vi "ExtendedKalmanFilter_SetXHat.vi"(10 "xHat":T1, 11 "in ExtendedKalmanFiilter":T2) -> (0 "Size Coerced":bool, 3 "out ExtendedKalmanFiilter":T2)   [LabVIEW 2019, in "Trajectory_Library.lvlib"]
doc: "Set initial state estimate x-hat.\n \nInputs:\n - inExtendedKalmanFIlter -- filter data cluster\n - xHat The state estimate x-hat.\n\nReturns:\n - outExtendedKalmanFIlter -- updated filter data cluster\n - sizeCoerced -- If TRUE, an unexpected error occured."
uses:
  Trajectory_Library.lvlib
  TypeDef/EXTENDED_KALMAN_FILTER.ctl
  <vilib>/Analysis/Matrix/Datatypes/RealMatrix.ctl
  MatBuilder_Create.vi
  <vilib>/Analysis/Matrix/NI_Matrix.lvlib
panel:
  # "State Estimate <Statess,1>"
  # "<States, States>"
  # "<States, States>"
  # "<Statess,  States>"
  # "<Outputs, Outputs>"
  # "State Estimate <Statess,1>"
  # "<States, States>"
  # "<States, States>"
  # "<Statess,  States>"
  # "<Outputs, Outputs>"
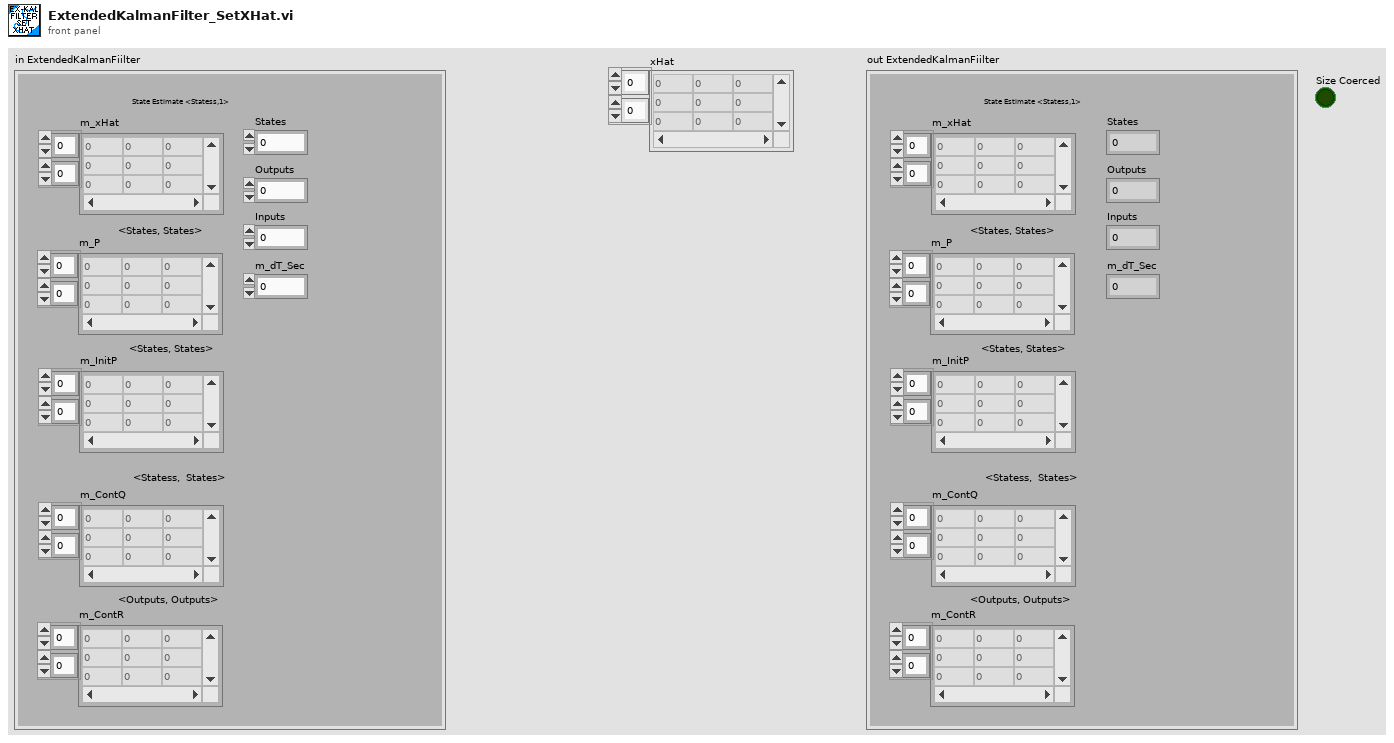
[diagram p1: front panel]
types:
  T1 = typedef "NI_Matrix.lvlib/RealMatrix.ctl" = dbl[][]
  T2 = typedef "Trajectory_Library.lvlib/EXTENDED_KALMAN_FILTER.ctl" = cluster{"m_P":T1, "m_xHat":T1, "States":i32, "Outputs":i32, "m_ContR":T1, "m_ContQ":T1, "m_dT_Sec":dbl, "Inputs":i32, "m_InitP":T1}
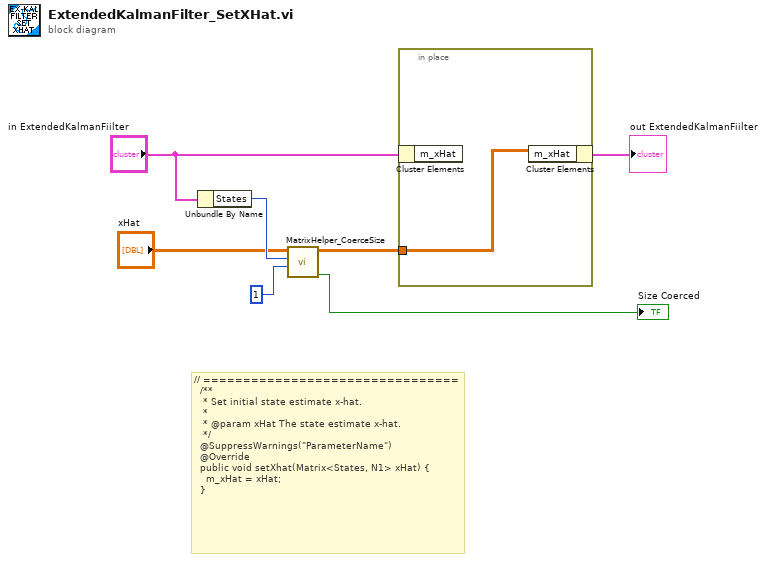
[diagram p0: block diagram]
diagram:
  # "// ================================\n  /**\n   * Set initial state estimate x-hat.\n   *\n   * @param xHat The state estimate x-hat.\n   */\n  @SuppressWarnings(\"ParameterName\")\n  @Override\n  public void setXhat(Matrix<States, N1> xHat) {\n    m_xHat = xHat;\n  }"
  n1 = Unbundle By Name("in ExtendedKalmanFiilter") -> ("States"=w6:i32)
  n2 = call "MatrixHelper_CoerceSize.vi"("Columns"=1, "Rows"=w6, "input matrix"="xHat") -> ("Coerced"=→"Size Coerced":bool, "output matrix"=w3:T1)  [unwired: 7 in]
  n3 = in-place {
    in-place-border: w3 -> [w8]
    n4 = in-place-cluster #1("in ExtendedKalmanFiilter") -> ()  [unwired: 1 out]
    n5 = in-place-cluster #1("m_xHat"=w8) -> (→"out ExtendedKalmanFiilter":T2)
  }
